vi "Write ITX (1D multi).vi"(0 "Commands":string, 5 "filename":path, 7 "Notes":string, 8 "1D Arrays Names":string[](array[string]), 9 "1D Arrays":dbl[][](array[numeric]), 10 "2D Array name":string, 11 "2D Array":dbl[][](array[numeric])) -> ()   [LabVIEW 2016, in "Data.ITX.lvclass"]
uses:
  Data.ITX.lvclass
panel:
  out "String":string
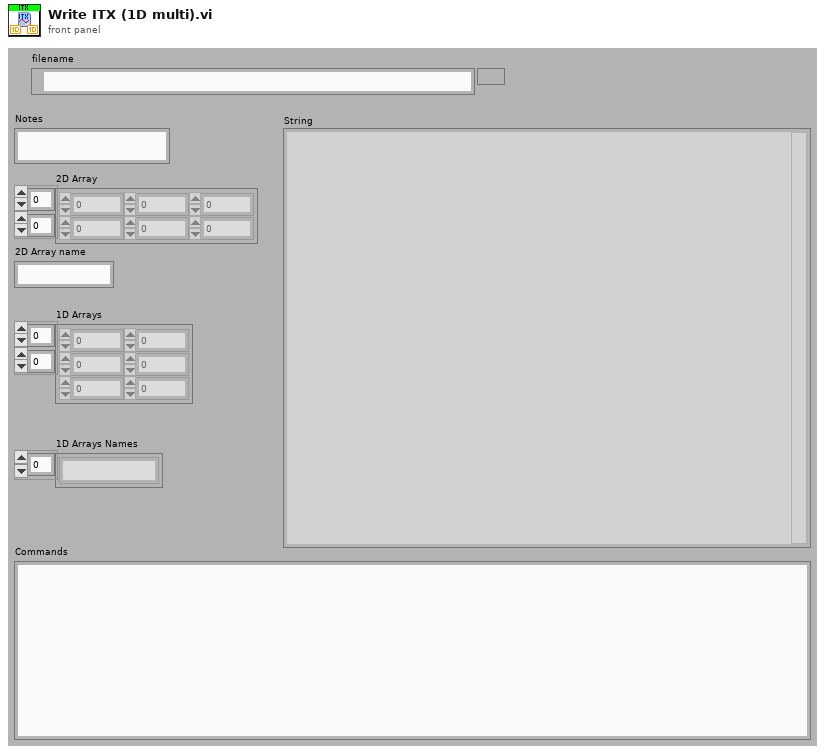
[diagram p1: front panel]
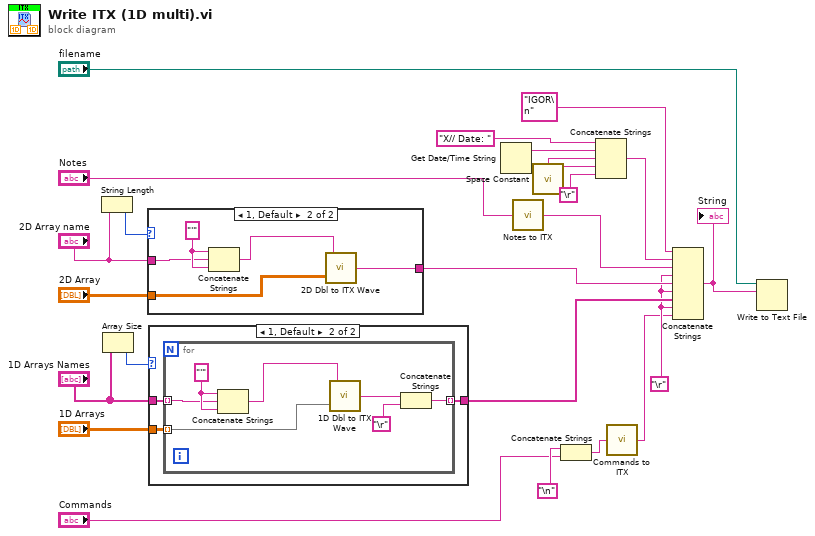
[diagram p0: block diagram]
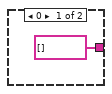
[diagram p2: hidden frame]
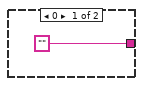
[diagram p3: hidden frame]
diagram:
  w12 = "\r"
  n1 = String Length(string="2D Array name") -> (length=w6:i32)
  n2 = Array Size(array="1D Arrays Names") -> (size(s)=w8:i32)
  n3 = case shown="1, Default" w6 {
    tunnel: ["" ("String") w29] -> w19
    tunnel: "2D Array name" -> [_ w27]
    tunnel: "2D Array" -> [_ w30]
    frame 0 {
    }
    frame 1, Default {
      w28 = "'"
      n4 = Concatenate Strings(w28, w27, w28) -> (w26:string)
      n5 = call "2D Dbl to ITX Wave.vi"("2D Array"=w30, "Wavename"=w26) -> ("ITX Wave"=w29:string)
    }
  }
  n6 = case shown="1, Default" w8 {
    tunnel: "1D Arrays Names" -> [_ w34]
    tunnel: "1D Arrays" -> [_ w33]
    tunnel: [string[] [] w32] -> w15
    frame 0 {
    }
    frame 1, Default {
      n7 = for {
        tunnel: [w41] -> w32 mode=indexing
        tunnel: w34 -> [w36] mode=indexing
        tunnel: w33 -> [w39] mode=indexing
        w37 = "'"
        n8 = Concatenate Strings(w37, w36, w37) -> (w35:string)
        n9 = call "1D Dbl to ITX Wave.vi"("1D Array"=w39, "Wavename"=w35) -> ("ITX Wave"=w38:string)
        n10 = Concatenate Strings(w38, "\r") -> (w41:string)
      }
    }
  }
  n11 = Get Date/Time String() -> (date string=w23:string, time string=w24:string)  [unwired: 3 out]
  n12 = call "Notes to ITX.vi"("Notes"="Notes") -> ("ITX Notes"=w3:string)
  n13 = call <vilib>:"Space Constant.vi"() -> ("String"=w18:string)
  n14 = Concatenate Strings("\n", "Commands") -> (w5:string)
  n15 = Concatenate Strings("X// Date: " ("format string"), w23, w18, w24, "\r") -> (w22:string)
  n16 = call "Commands to ITX.vi"("Commands"=w5) -> ("ITX Commands"=w4:string)
  n17 = Concatenate Strings("IGOR\n", w22, w3, w12, w19, w12, w15, w12, w4) -> (w14:string)
  "String" <- w14
  n18 = Write to Text File(file (use dialog)="filename", text=w14) -> ()  [unwired: 1 in, 4 out]
